vi "Initialize_ErrorHandler.vi"(8 "error in (no error)":errorcluster) -> (0 "error out":errorcluster, 3 "ErrorHandler out":refnum<class "ErrorHandler.lvclass">)   [LabVIEW 2019, in "ErrorHandler.lvclass"]
doc: "Developed by Kevin Thompson\nkevin@thompsonengineering.net\n\nCopyright 2018\nThompson Engineering, LLC"
uses:
  ErrorHandler.lvclass
  TypeDef/ErrorRemote EventData.ctl
  TypeDef/ObjData--cluster.ctl
  TypeDef/TD GetSet ActionSelect--enum.ctl
  TypeDef/Public Events.ctl
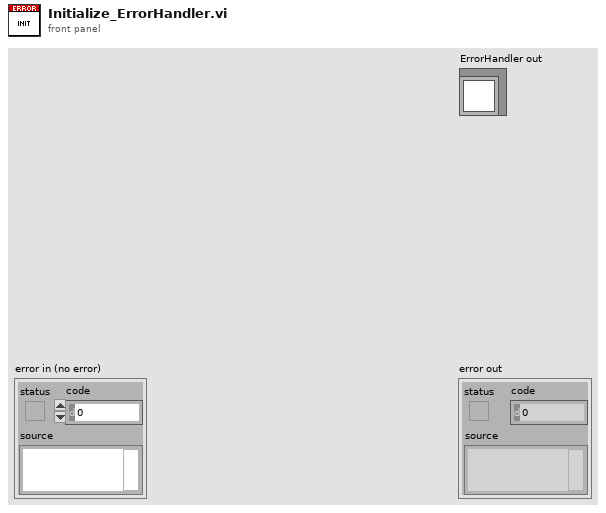
[diagram p1: front panel]
types:
  T1 = typedef "ErrorHandler.lvclass/TD GetSet ActionSelect--enum.ctl" = enum16{"Init", "Get", "Set"}
  T2 = typedef "ErrorHandler.lvclass/ObjData--cluster.ctl" = cluster{"AppName":string, "ErrorLogBasePath":path, "ErrorDialogPopUp Disabled":bool, "TerminateAppOnError Enabled":bool, "Public Events":T3, "ErrorList Qref":refnum<queue>}
  T3 = typedef "ErrorHandler.lvclass/Public Events.ctl" = cluster{"ErrorRemote Ev":refnum<user-event>}
  T4 = typedef "ErrorHandler.lvclass/ErrorRemote EventData.ctl" = cluster{"Timestamp":timestamp, "ErrorCluster":errorcluster, "message":string, "Shutdown?":bool, "DialogDisabled?":bool, "TerminateOnError?":bool}
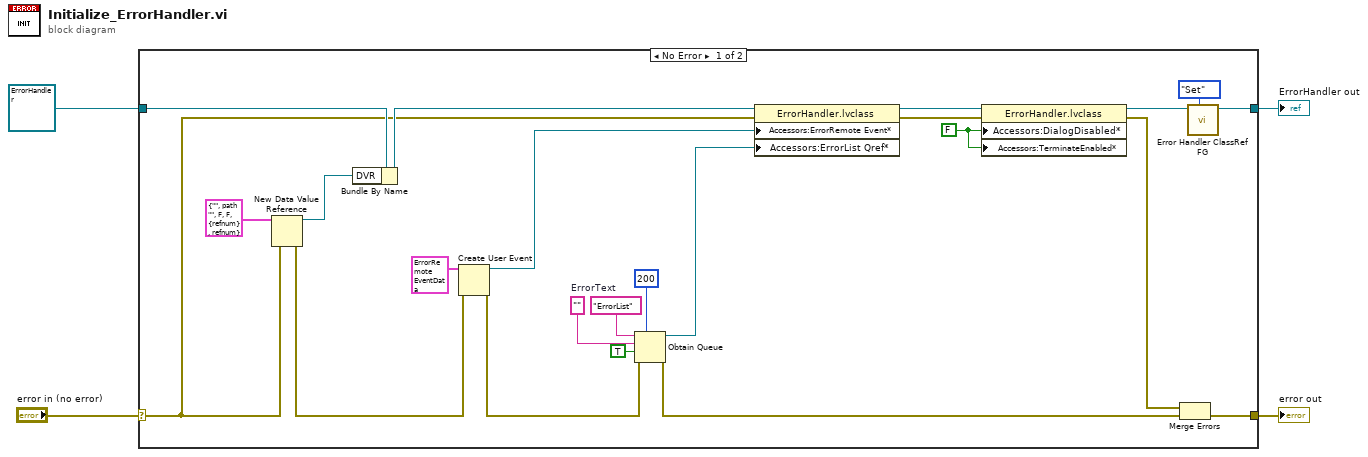
[diagram p0: block diagram]
diagram:
  n1 = case shown="No Error" "error in (no error)" {
    selector: "error in (no error)" -> [w7 w29]
    tunnel: [w15 w29] -> w3
    tunnel: [w11 w28] -> w1
    tunnel: refnum<class "ErrorHandler.lvclass"> refnum ("ErrorHandler in") -> [w27 w28]
    frame No Error {
      w16 = FALSE ("DialogEnabled*")
      w25 = ""  # ErrorText
      n2 = New Data Value Reference(data value=T2 {"AppName"="", "ErrorLogBasePath"=path "", "ErrorDialogPopUp Disabled"=FALSE, "TerminateAppOnError Enabled"=FALSE, "Public Events"={"ErrorRemote Ev"=refnum}, "ErrorList Qref"=refnum} ("ObjData"), error in=w7) -> (data value reference=w20:refnum<data-value>, error out=w21:errorcluster)
      n3 = Bundle By Name(cluster=w27, "DVR"=w20) -> (w17:refnum<class "ErrorHandler.lvclass">)
      n4 = Create User Event(user event datatype=T4 {"Timestamp"=timestamp(0 s since 1904-01-01), "ErrorCluster"={"status"=FALSE, "code"=0, "source"=""}, "message"="", "Shutdown?"=FALSE, "DialogDisabled?"=FALSE, "TerminateOnError?"=FALSE} ("ErrorRemote"), error in=w21) -> (user event=w8:refnum<user-event>, error out=w22:errorcluster)
      n5 = Obtain Queue(max queue size (-1, unlimited)=200, name (unnamed)="ErrorList", element data type=w25, create if not found? (T)=TRUE, error in (no error)=w22) -> (queue out=w9:refnum<queue>, error out=w6:errorcluster)  [unwired: 1 out]
      n6 = property class="ErrorHandler.lvclass"(reference=w17, error in=w7, "Accessors:ErrorRemote Event*"=w8, "Accessors:ErrorList Qref*"=w9) -> (reference out=w10:refnum<class "ErrorHandler.lvclass">, error out=w5:errorcluster)
      n7 = property class="ErrorHandler.lvclass"(reference=w10, error in=w5, "Accessors:DialogDisabled*"=w16, "Accessors:TerminateEnabled*"=w16) -> (reference out=w12:refnum<class "ErrorHandler.lvclass">, error out=w14:errorcluster)
      n8 = Merge Errors(w14, w6) -> (w15:errorcluster)
      n9 = call "Error Handler ClassRef FG.vi"("action (Get)"=TD_GetSet_ActionSelect--enum."Set", "ErrorHandler in"=w12) -> ("ErrorHandler out"=w11:refnum<class "ErrorHandler.lvclass">)  [unwired: 8 in, 1 out]
    }
    frame Error {
    }
  }
  "error out" <- w3
  "ErrorHandler out" <- w1
